vi "Auto settings.vi"(8 "error in (no error)":errorcluster, 10 "Component Tray Settings":T1, 11 "Component Tray in":refnum<class "Component Tray.lvclass">) -> (0 "error out":errorcluster, 3 "Component Tray out":refnum<class "Component Tray.lvclass">)   [LabVIEW 2021, in "Component Tray.lvclass"]
uses:
  Component Tray.lvclass
  C:/Users/HEP/Documents/GitHub/Gantry/UCSB-Gantry-HEP-main/Classes/Workspace/Fixture.lvclass
  Component Tray.lvclass/Component Tray.ctl
  Fixture.lvclass/Fixture.ctl
  Write Gantry Region.vi
  Write Fixture ID.vi
  Write Position.vi
  SubVIs/component_tray_region.vi
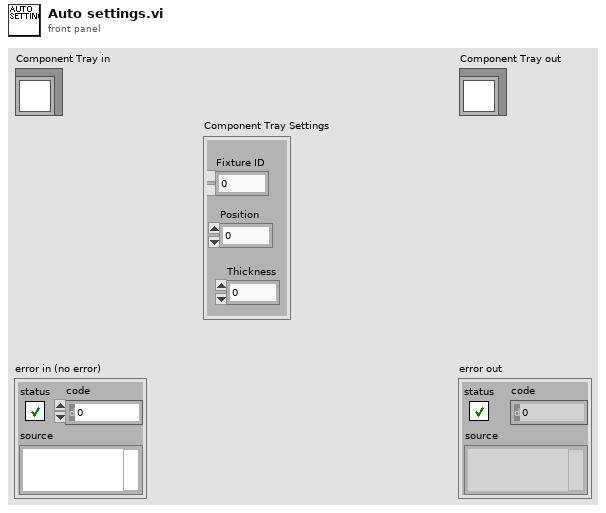
[diagram p1: front panel]
types:
  T1 = cluster{"Fixture ID":dbl, "Position":dbl, "Thickness":dbl}
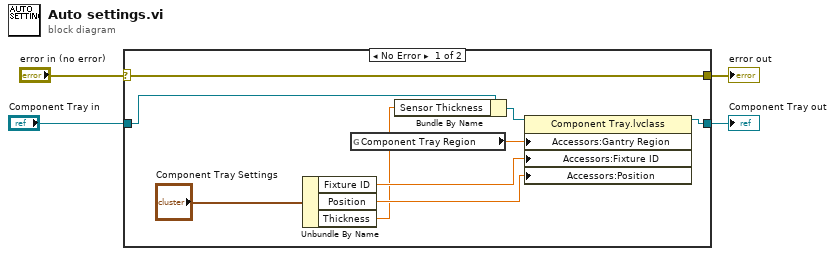
[diagram p0: block diagram]
diagram:
  n1 = case shown="No Error" "error in (no error)" {
    selector: "error in (no error)" -> [w13 w15]
    tunnel: [w13 w15] -> w3
    tunnel: [w12 w14] -> w1
    tunnel: "Component Tray in" -> [w7 w14]
    frame No Error {
      n2 = Unbundle By Name("Component Tray Settings") -> ("Fixture ID"=w9:dbl, "Position"=w8:dbl, "Thickness"=w6:dbl)
      n3 = global read "component_tray_region.vi" "Component Tray Region"() -> (w11:dbl)
      n4 = Bundle By Name(cluster=w7, "Sensor Thickness"=w6) -> (w5:refnum<class "Component Tray.lvclass">)
      n5 = property class="Component Tray.lvclass"(reference=w5, "Accessors:Gantry Region"=w11, "Accessors:Fixture ID"=w9, "Accessors:Position"=w8) -> (reference out=w12:refnum<class "Component Tray.lvclass">)  [unwired: 1 in, 1 out]
    }
    frame Error {
    }
  }
  "error out" <- w3
  "Component Tray out" <- w1
